vi "Upload to Sift.vi"(6 "API REST URL":string, 7 "Absolute Filepath":path, 8 "Run Name":string="TDMS Upload Example", 9 "Asset Name":string="LabVIEW-TDMS-Example", 10 "API Key":string, 11 "API GRPC URL":string) -> (0 "Error":errorcluster, 3 "Run URL":string)   [LabVIEW 2024, in "Sift TDMS Uploader.lvlib" / "Sift TDMS Uploader.lvclass"]
uses:
  Sift TDMS Uploader.lvclass
  <vilib>/Sift/Sift/Sift API/Sift Client.lvclass
  Sift TDMS Uploader.lvclass/Sift TDMS Uploader.ctl
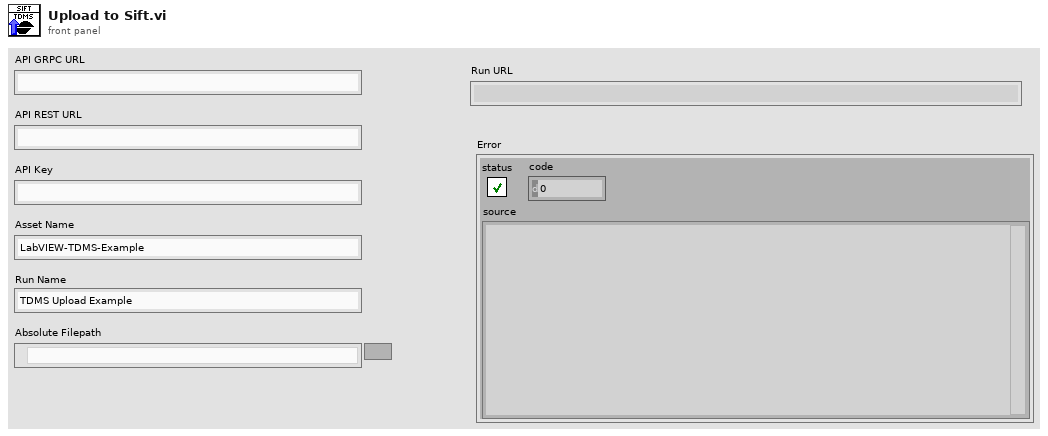
[diagram p1: front panel]
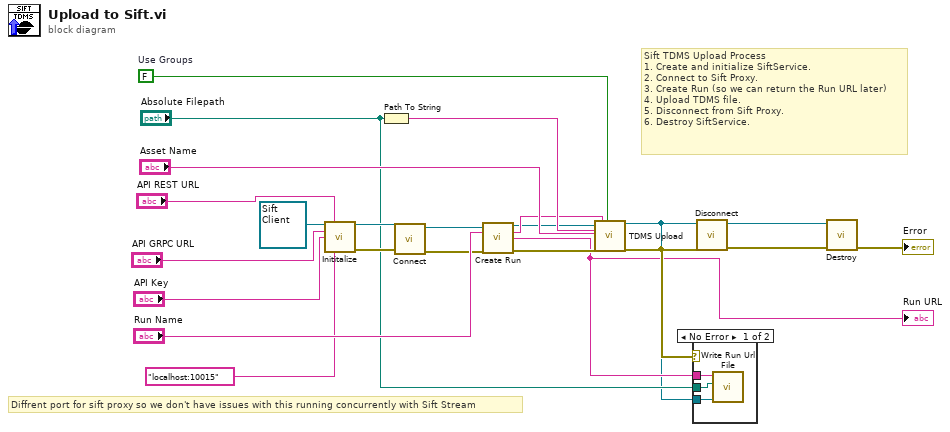
[diagram p0: block diagram]
diagram:
  w16 = FALSE  # Use Groups
  # "Diffrent port for sift proxy so we don't have issues with this running concurrently with Sift Stream"
  # "Sift TDMS Upload Process\n1. Create and initialize SiftService.\n2. Connect to Sift Proxy.\n3. Create Run (so we can return the Run URL later)\n4. Upload TDMS file.\n5. Disconnect from Sift Proxy.\n6. Destroy SiftService."
  n1 = call-dynamic "Inititalize.vi"("Sift Client in"=refnum<class "Sift Client.lvclass"> refnum ("Sift Client.lvlib:Sift Client.lvclass"), "REST URL"="API REST URL", "GRPC URL"="API GRPC URL", "API Key"="API Key", "Sift Proxy Address"="localhost:10015") -> ("Sift Client out"=w21:refnum<class "Sift Client.lvclass">, "error out"=w15:errorcluster)  [unwired: 9 in]
  n2 = Path To String(path="Absolute Filepath") -> (string=w17:string)
  n3 = call-dynamic "Connect.vi"("error in (no error)"=w15, "Sift Client in"=w21) -> ("error out"=w10:errorcluster, "Sift Client out"=w7:refnum<class "Sift Client.lvclass">)  [unwired: 7 in, 1 out]
  n4 = call-dynamic "Create Run.vi"("Sift Client in"=w7, "Name"="Run Name", "error in (no error)"=w10) -> ("Sift Client out"=w6:refnum<class "Sift Client.lvclass">, "Run ID"=w8:string, "URL"=w2:string, "error out"=w9:errorcluster)  [unwired: 9 in]
  "Run URL" <- w2
  n5 = call-dynamic "TDMS Upload.vi"("Sift Client in"=w6, "Filepath"=w17, "Asset Name"="Asset Name", "error in (no error)"=w9, "Run ID"=w8, "Group Into Components"=w16) -> ("Sift Client out"=w1:refnum<class "Sift Client.lvclass">, "error out"=w4:errorcluster)  [unwired: 12 in]
  n6 = case shown="No Error" w4 {
    tunnel: "Absolute Filepath" -> [w26 _]
    tunnel: w2 -> [w25 _]
    tunnel: w1 -> [w24 _]
    frame No Error {
      n7 = call "Write Run Url File.vi"("Sift Client in"=w24, "TDMS Filepath"=w26, "Run URL"=w25) -> ()  [unwired: 9 in]
    }
    frame Error {
    }
  }
  n8 = call-dynamic "Disconnect.vi"("error in (no error)"=w4, "Sift Client in"=w1) -> ("error out"=w19:errorcluster, "Sift Client out"=w20:refnum<class "Sift Client.lvclass">)  [unwired: 8 in]
  n9 = call-dynamic "Destroy.vi"("error in (no error)"=w19, "Sift Client in"=w20) -> ("error out"=→"Error":errorcluster)  [unwired: 8 in, 1 out]
